vi "Test - copia2.vi"() -> ()   [LabVIEW 2010]
panel:
  in  "String 2":string="/COLAB/JiLTest"
  in  "Vi to open":T1(ring)
  in  "stringin":string
  in  "booleanin":bool=TRUE
  in  "doublein":dbl
  in  "intin":i32
  in  "Mensajes":T2(ring)
  in  "stop":bool
  in  "Send":bool=TRUE
  out "error out":errorcluster
  out "Respuesta":string
  out "Mensaje":string
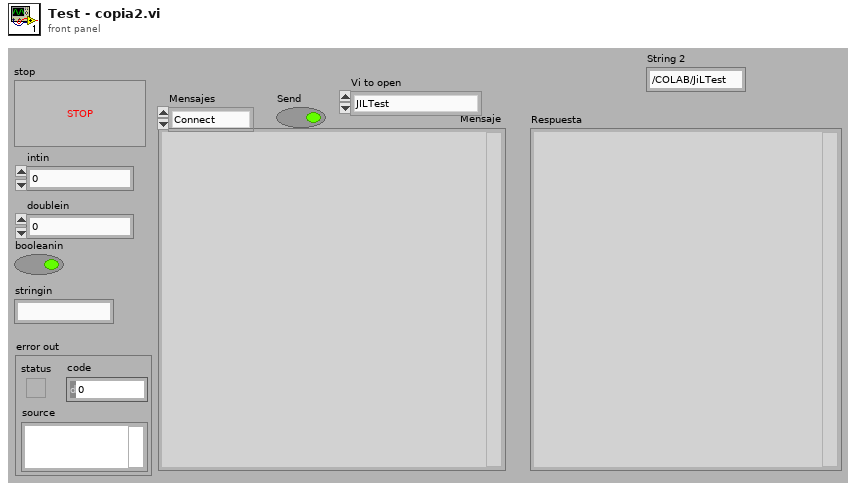
[diagram p1: front panel]
types:
  T1 = enum16{"JILTest", "/COLAB/JiLTest", "/COLAB/JiLTestR", "JILTest2", "JILTestR"}
  T2 = enum16{"Connect", "OpenVi", "SyncVi", "RunVi", "StopVi", "CloseVi", "Disconnect"}
  T3 = enum16{"Standard", "Buffered", "CRLF", "Immediate"}
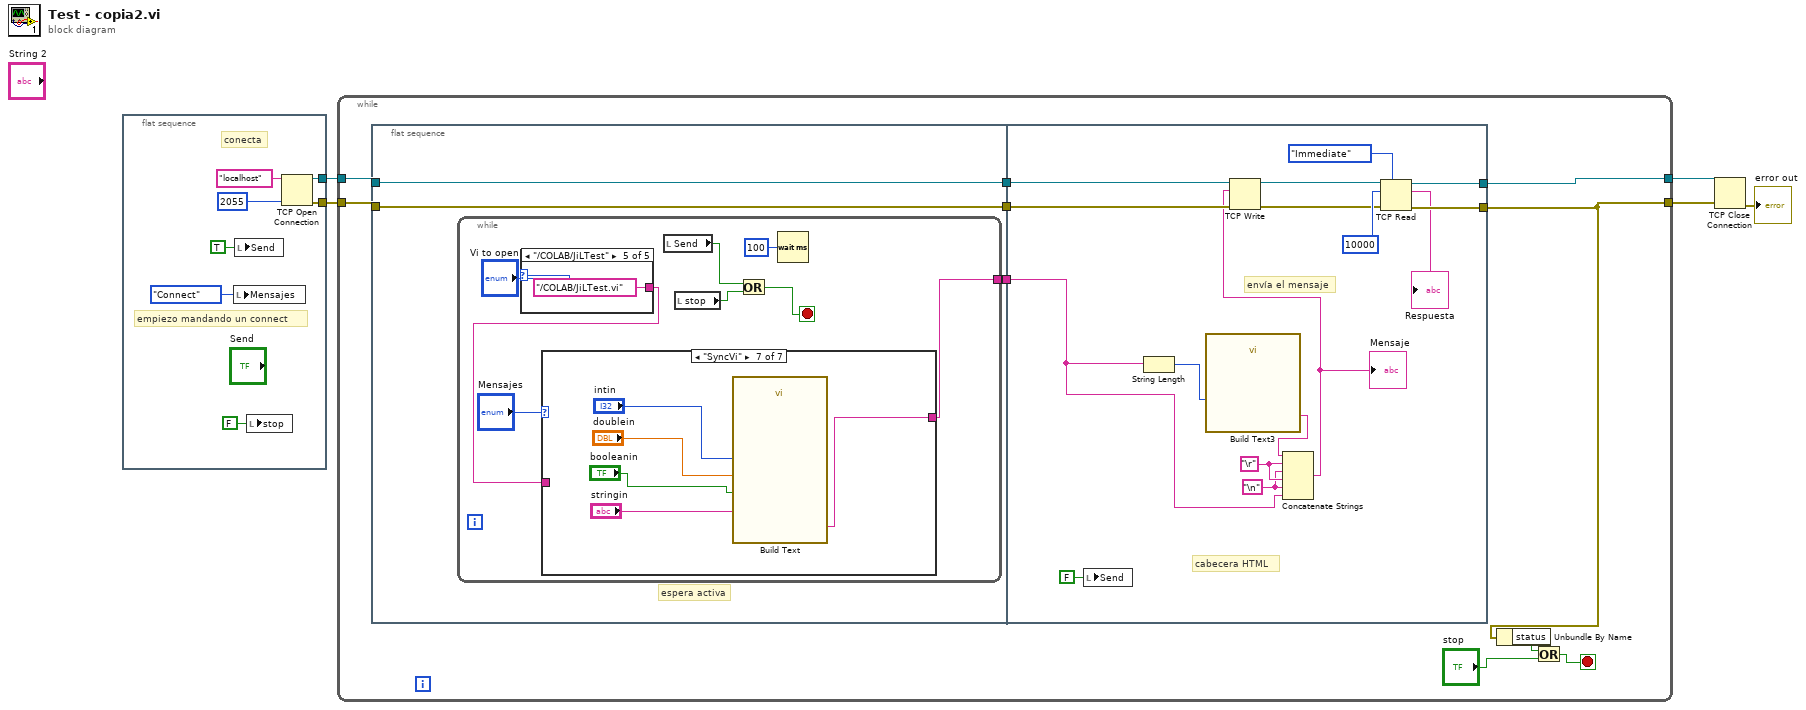
[diagram p0: block diagram]
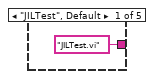
[diagram p2: hidden frame]
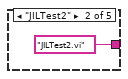
[diagram p3: hidden frame]
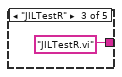
[diagram p4: hidden frame]
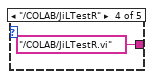
[diagram p5: hidden frame]
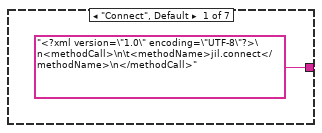
[diagram p6: hidden frame]
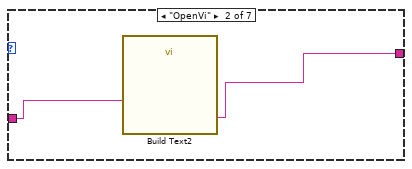
[diagram p7: hidden frame]
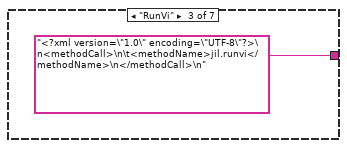
[diagram p8: hidden frame]
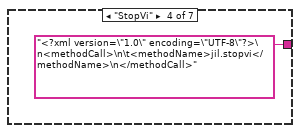
[diagram p9: hidden frame]
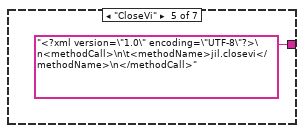
[diagram p10: hidden frame]
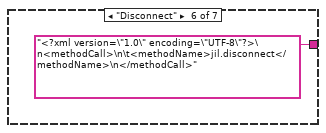
[diagram p11: hidden frame]
diagram:
  n1 = flat-sequence {
    tunnel: [w10] -> w5
    tunnel: [w9] -> w4
    frame #0 {
      # "empiezo mandando un connect"
      # "conecta"
      n2 = local write "Mensajes"(T2."Connect" ("Mensajes")) -> ()
      n3 = local write "Send"(TRUE ("Send")) -> ()
      n4 = local write "stop"(FALSE ("stop")) -> ()
      n5 = TCP Open Connection(address="localhost", remote port or service name=u16 2055) -> (connection ID=w10:refnum<k5>, error out=w9:errorcluster)  [unwired: 3 in]
    }
  }
  n6 = while {
    tunnel: w5 -> [w20]
    tunnel: w4 -> [w19]
    tunnel: [w18] -> w2
    tunnel: [w15] -> w1
    stop <- w16 stop-if-true
    n7 = flat-sequence {
      tunnel: [w25] -> w22
      tunnel: [w24] -> w21
      tunnel: [w23] -> w13
      tunnel: w19 -> [w25]
      tunnel: w20 -> [w24]
      tunnel: [w64] -> w18
      tunnel: [w63] -> w15
      tunnel: w22 -> [w62]
      tunnel: w21 -> [w61]
      tunnel: w13 -> [w54]
      frame #0 {
        # "espera activa"
        n8 = while {
          tunnel: [w28] -> w23
          stop <- w32 stop-if-true
          n9 = case shown="\"/COLAB/JiLTest\"" "Vi to open" {
            tunnel: ["JILTest.vi" "JILTest2.vi" "JILTestR.vi" "/COLAB/JiLTestR.vi" "/COLAB/JiLTest.vi"] -> w26
            frame "JILTest", Default {
            }
            frame "JILTest2" {
            }
            frame "JILTestR" {
            }
            frame "/COLAB/JiLTestR" {
            }
            frame "/COLAB/JiLTest" {
            }
          }
          n10 = case shown="\"SyncVi\"" "Mensajes" {
            tunnel: ["<?xml version=\"1.0\" encoding=\"UTF-8\"?>\n<methodCall>\n\t<methodName>jil.connect</methodName>\n</methodCall>" w40 "<?xml version=\"1.0\" encoding=\"UTF-8\"?>\n<methodCall>\n\t<methodName>jil.runvi</methodName>\n</methodCall>\n" "<?xml version=\"1.0\" encoding=\"UTF-8\"?>\n<methodCall>\n\t<methodName>jil.stopvi</methodName>\n</methodCall>" "<?xml version=\"1.0\" encoding=\"UTF-8\"?>\n<methodCall>\n\t<methodName>jil.closevi</methodName>\n</methodCall>" "<?xml version=\"1.0\" encoding=\"UTF-8\"?>\n<methodCall>\n\t<methodName>jil.disconnect</methodName>\n</methodCall>" w50] -> w28
            tunnel: w26 -> [_ w41 _ _ _ _ _]
            frame "Connect", Default {
            }
            frame "OpenVi" {
              n11 = call "Build Text2"("name"=w41) -> ("Result"=w40:string)  [unwired: 13 in, 1 out]
            }
            frame "RunVi" {
            }
            frame "StopVi" {
            }
            frame "CloseVi" {
            }
            frame "Disconnect" {
            }
            frame "SyncVi" {
              n12 = call "Build Text"("string"="stringin", "int"="intin", "double"="doublein", "bolean"="booleanin") -> ("Result"=w50:string)  [unwired: 10 in, 1 out]
            }
          }
          n13 = local read "Send"() -> (w30:bool)
          n14 = local read "stop"() -> (w31:bool)
          n15 = Or(x=w30, y=w31) -> (x .or. y?=w32:bool)
          n16 = Wait (ms)(milliseconds to wait=u32 100) -> ()  [unwired: 1 out]
        }
      }
      frame #1 {
        w55 = "\n"
        w56 = "\r"
        # "cabecera HTML"
        # "envía el mensaje"
        n17 = local write "Send"(FALSE ("Send")) -> ()
        n18 = String Length(string=w54) -> (length=w58:i32)
        n19 = call "Build Text3"("longitud"=w58) -> ("Result"=w57:string)  [unwired: 13 in, 1 out]
        n20 = Concatenate Strings(w57, w56, w55, w56, w55, w54) -> (w51:string)
        "Mensaje" <- w51
        n21 = TCP Write(connection ID=w61, data in=w51, error in (no error)=w62) -> (connection ID out=w53:refnum<k5>, error out=w52:errorcluster)  [unwired: 1 in, 1 out]
        n22 = TCP Read(connection ID=w53, bytes to read=10000, error in (no error)=w52, 7:T3."Immediate" ("mode (standard)")) -> (connection ID out=w64:refnum<k5>, data out=→"Respuesta":string, error out=w63:errorcluster)  [unwired: 1 in]
      }
    }
    n23 = Unbundle By Name(w15) -> ("status"=w14:bool)
    n24 = Or(x=w14, y="stop") -> (x .or. y?=w16:bool)
  }
  n25 = TCP Close Connection(connection ID=w2, error in (no error)=w1) -> (error out=→"error out":errorcluster)  [unwired: 1 in, 1 out]
